vi "GEOM_VAR_Constants.vi"(9 "Action":T1, 10 "GEOM_constants":string[][](table)) -> (2 "GEOM_constants out":string[][](table))   [LabVIEW 2016]
uses:
  GEOM_VAR_action.ctl
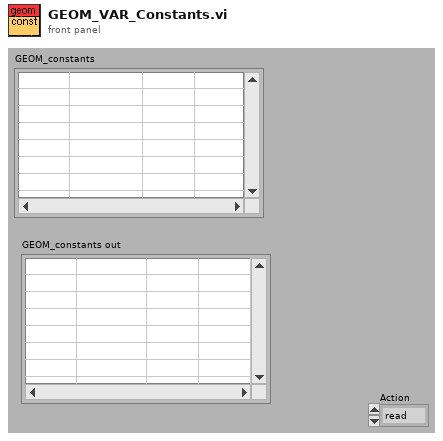
[diagram p1: front panel]
types:
  T1 = typedef "GEOM_VAR_action.ctl" = enum16{"read", "write"}
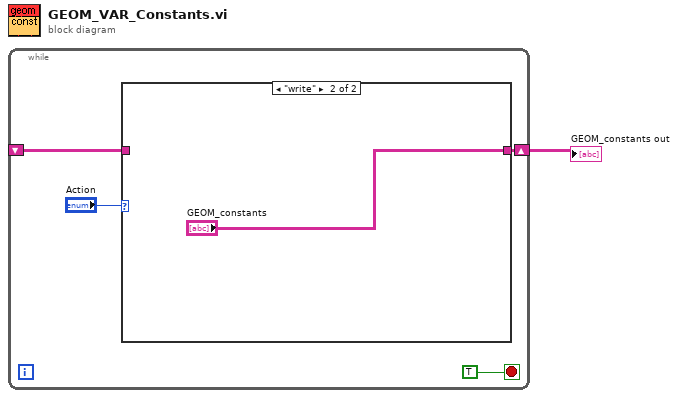
[diagram p0: block diagram]
diagram:
  n1 = while {
    shift-right: [w4] -> w1
    shift-left: _ -> [w3]
    stop <- TRUE stop-if-true
    n2 = case shown="\"write\"" "Action" {
      tunnel: [w6 "GEOM_constants"] -> w4
      tunnel: w3 -> [w6 _]
      frame "read", Default {
      }
      frame "write" {
      }
    }
  }
  "GEOM_constants out" <- w1
